vi "Redo.vi"(8 "error in":errorcluster, 11 "History in":refnum<class "History.lvclass">) -> (0 "error out":errorcluster, 2 "State":string, 3 "History out":refnum<class "History.lvclass">)   [LabVIEW 2020, in "lv_icon.lvlib" / "History.lvlib" / "History.lvclass"]
doc: "Gets the next state so than a Redo action may be performed."
uses:
  History.lvclass
  History.lvclass/History.ctl
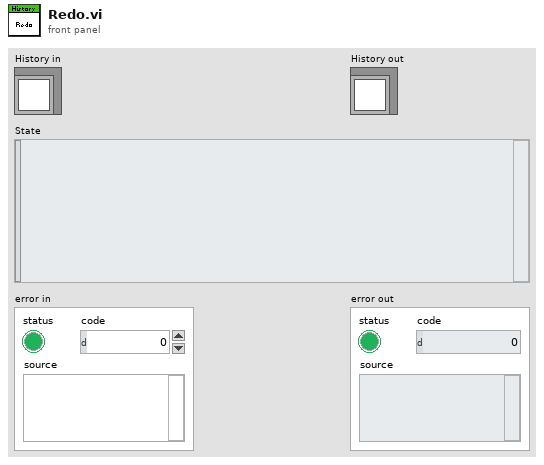
[diagram p1: front panel]
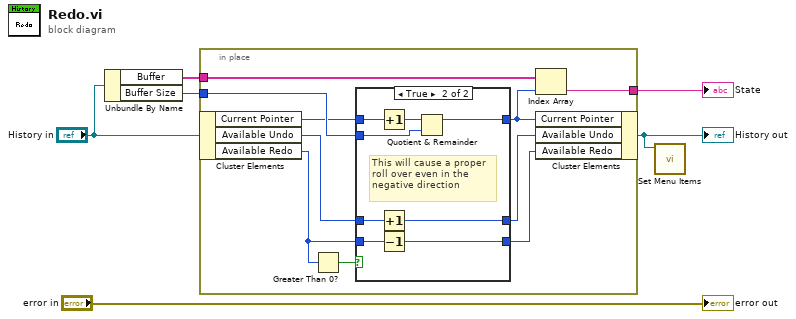
[diagram p0: block diagram]
diagram:
  n1 = Unbundle By Name("History in") -> ("Buffer"=w5:string[], "Buffer Size"=w4:i32)
  n2 = in-place {
    in-place-border: w5 -> [w11]
    in-place-border: w4 -> [w16]
    in-place-border: [w7] -> w2
    n3 = in-place-cluster #1("History in") -> ("Current Pointer"=w12:i32, "Available Undo"=w14:i32, "Available Redo"=w13:i32)
    n4 = Greater Than 0?(x=w13) -> (x > 0?=w15:bool)
    n5 = case shown="True" w15 {
      tunnel: w12 -> [w19 w22]
      tunnel: [w19 w20] -> w10
      tunnel: w16 -> [_ w27]
      tunnel: w14 -> [w18 w26]
      tunnel: [w18 w25] -> w9
      tunnel: w13 -> [w17 w24]
      tunnel: [w17 w23] -> w8
      frame False {
      }
      frame True {
        # "This will cause a proper\nroll over even in the\nnegative direction"
        n6 = Increment(x=w22) -> (x+1=w21:i32)
        n7 = Increment(x=w26) -> (x+1=w25:i32)
        n8 = Decrement(x=w24) -> (x-1=w23:i32)
        n9 = Quotient & Remainder(x=w21, y=w27) -> (x-y*floor(x/y)=w20:i32)  [unwired: 1 out]
      }
    }
    n10 = Index Array(array=w11, index=w10) -> (element=w7:string)
    n11 = in-place-cluster #1("Current Pointer"=w10, "Available Undo"=w9, "Available Redo"=w8) -> (w3:refnum<class "History.lvclass">)
  }
  "History out" <- w3
  "State" <- w2
  n12 = call "Set Menu Items.vi"("History"=w3) -> ()  [unwired: 11 in]
  "error out" <- "error in"
